vi "FPGA_CounterWriteTimerConfiguration.vi"(6 "UpdateWhenEmpty":bool=TRUE, 8 "error in (no error)":errorcluster, 9 "Average Size":u8=1, 10 "StallPeriod (s)":dbl=0.05, 11 "Ctr Ref in":T1={"DevStatus"={"status"=FALSE, "code"=0, "source"=""}, "CntIndex"=enum."Ctr 1"}) -> (0 "error out":errorcluster, 3 "Ctr Ref out":T1={"DevStatus"={"status"=FALSE, "code"=0, "source"=""}, "CntIndex"=enum."Ctr 1"})   [LabVIEW 2017]
uses:
  <vilib>/Rock Robotics/SystemInterfaces/Counter/FPGA_CounterCtrDevRef.ctl
  <vilib>/Rock Robotics/SystemInterfaces/Counter/FPGA_CounterCtrSystemIndex.ctl
  <vilib>/Rock Robotics/SystemInterfaces/System/FPGA_SystemFPGA Ref Global.vi
  <vilib>/Utility/error.llb/Error Cluster From Error Code.vi
  <vilib>/rvi/errors/niLvFpgaAdjustHostInterfaceError.vi
  <vilib>/rvi/interface/nirviReadWriteControl/nirviReadWriteControl.xnode
  <vilib>/Rock Robotics/SystemInterfaces/System/FPGA_SystemFRC FPGA Ref.ctl
  NiFpgaLv.dll
  <vilib>/rvi/interface/Simulation/niFpgaSimulationCallBeginRW.vi
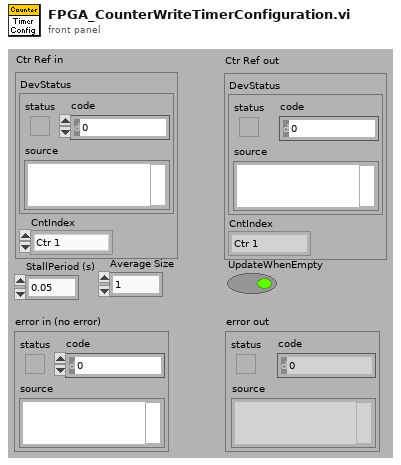
[diagram p1: front panel]
types:
  T1 = typedef "FPGA_CounterCtrDevRef.ctl" = cluster{"DevStatus":errorcluster, "CntIndex":T2}
  T2 = typedef "FPGA_CounterCtrSystemIndex.ctl" = enum8{"Ctr 0", "Ctr 1", "Ctr 2", "Ctr 3", "Ctr 4", "Ctr 5", "Ctr 6", "Ctr 7", "Invalid"}
  T3 = typedef "FPGA_SystemFRC FPGA Ref.ctl" = refnum<k20>
  T4 = cluster{"StallPeriod":fxp<+,24,25>, "AverageSize":fxp<+,7,7>, "UpdateWhenEmpty":bool}
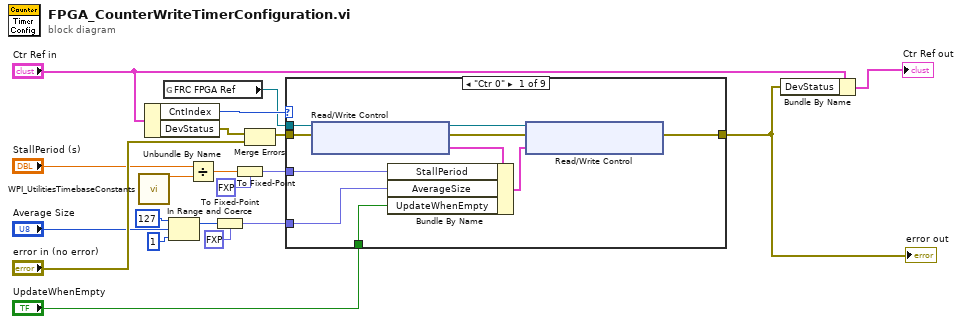
[diagram p0: block diagram]
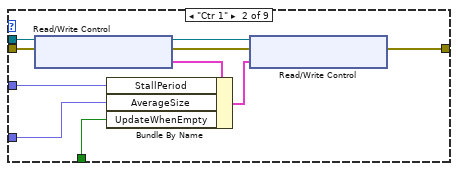
[diagram p2: hidden frame]
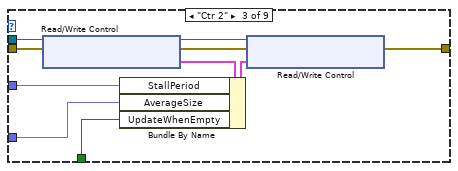
[diagram p3: hidden frame]
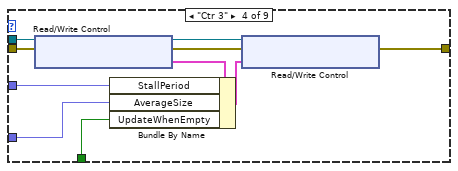
[diagram p4: hidden frame]
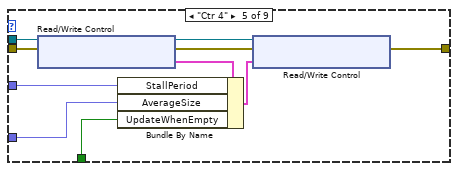
[diagram p5: hidden frame]
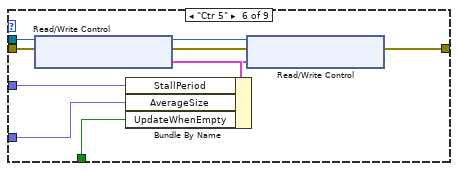
[diagram p6: hidden frame]
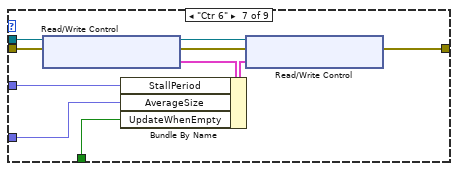
[diagram p7: hidden frame]
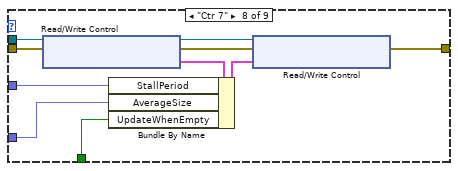
[diagram p8: hidden frame]
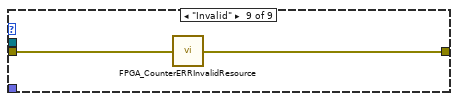
[diagram p9: hidden frame]
diagram:
  n1 = call <vilib>:"WPI_UtilitiesTimebaseConstants.vi"() -> ("40 MHz FPGA clock"=w1:dbl)  [unwired: 13 in, 2 out]
  n2 = Unbundle By Name("Ctr Ref in") -> ("CntIndex"=w14:T2, "DevStatus"=w4:errorcluster)
  n3 = global read "FPGA_SystemFPGA Ref Global.vi" "FRC FPGA Ref"() -> (w3:T3)
  n4 = In Range and Coerce(upper limit=u8 127, x="Average Size", lower limit=u8 1) -> (coerced(x)=w9:u8)  [unwired: 1 out]
  n5 = Divide(x="StallPeriod (s)", y=w1) -> (x/y=w13:dbl)
  n6 = To Fixed-Point(fixed-point type=fxp<+,7,7> 0.0 ("AverageSize"), number=w9) -> (fixed-point=w8:fxp<+,7,7>)
  n7 = To Fixed-Point(fixed-point type=fxp<+,24,25> 0.0 ("StallPeriod"), number=w13) -> (fixed-point=w12:fxp<+,24,25>)
  n8 = Merge Errors(w4, "error in (no error)") -> (w5:errorcluster)
  n9 = case shown="\"Ctr 0\"" w14 {
    tunnel: w3 -> [w21 w31 w50 w60 w70 w80 w90 w100 _]
    tunnel: w5 -> [w30 w34 w49 w59 w69 w77 w89 w99 w101]
    tunnel: [w27 w38 w46 w56 w66 w76 w86 w96 w102] -> w17
    tunnel: w12 -> [w24 w35 w45 w53 w64 w73 w83 w93 _]
    tunnel: w8 -> [w22 w32 w41 w51 w61 w71 w81 w92 _]
    tunnel: "UpdateWhenEmpty" -> [w23 w33 w42 w52 w62 w72 w82 w91 _]
    frame "Ctr 0" {
      n10 = xnode "Read/Write Control"("FPGA VI Reference In"=w21, "error in"=w30) -> ("FPGA VI Reference Out"=w28:T3, "error out"=w29:errorcluster, "Counter0.TimerConfig"=w26:T4)
      n11 = Bundle By Name(cluster=w26, "StallPeriod"=w24, "AverageSize"=w22, "UpdateWhenEmpty"=w23) -> (w25:T4)
      n12 = xnode "Read/Write Control"("FPGA VI Reference In"=w28, "error in"=w29, "Counter0.TimerConfig"=w25) -> ("error out"=w27:errorcluster)  [unwired: 1 out]
    }
    frame "Ctr 1" {
      n13 = xnode "Read/Write Control"("FPGA VI Reference In"=w31, "error in"=w34) -> ("FPGA VI Reference Out"=w39:T3, "error out"=w40:errorcluster, "Counter1.TimerConfig"=w37:T4)
      n14 = Bundle By Name(cluster=w37, "StallPeriod"=w35, "AverageSize"=w32, "UpdateWhenEmpty"=w33) -> (w36:T4)
      n15 = xnode "Read/Write Control"("FPGA VI Reference In"=w39, "error in"=w40, "Counter1.TimerConfig"=w36) -> ("error out"=w38:errorcluster)  [unwired: 1 out]
    }
    frame "Ctr 2" {
      n16 = xnode "Read/Write Control"("FPGA VI Reference In"=w50, "error in"=w49) -> ("FPGA VI Reference Out"=w48:T3, "error out"=w47:errorcluster, "Counter2.TimerConfig"=w44:T4)
      n17 = Bundle By Name(cluster=w44, "StallPeriod"=w45, "AverageSize"=w41, "UpdateWhenEmpty"=w42) -> (w43:T4)
      n18 = xnode "Read/Write Control"("FPGA VI Reference In"=w48, "error in"=w47, "Counter2.TimerConfig"=w43) -> ("error out"=w46:errorcluster)  [unwired: 1 out]
    }
    frame "Ctr 3" {
      n19 = xnode "Read/Write Control"("FPGA VI Reference In"=w60, "error in"=w59) -> ("FPGA VI Reference Out"=w57:T3, "error out"=w58:errorcluster, "Counter3.TimerConfig"=w55:T4)
      n20 = Bundle By Name(cluster=w55, "StallPeriod"=w53, "AverageSize"=w51, "UpdateWhenEmpty"=w52) -> (w54:T4)
      n21 = xnode "Read/Write Control"("FPGA VI Reference In"=w57, "error in"=w58, "Counter3.TimerConfig"=w54) -> ("error out"=w56:errorcluster)  [unwired: 1 out]
    }
    frame "Ctr 4" {
      n22 = xnode "Read/Write Control"("FPGA VI Reference In"=w70, "error in"=w69) -> ("FPGA VI Reference Out"=w67:T3, "error out"=w68:errorcluster, "Counter4.TimerConfig"=w65:T4)
      n23 = Bundle By Name(cluster=w65, "StallPeriod"=w64, "AverageSize"=w61, "UpdateWhenEmpty"=w62) -> (w63:T4)
      n24 = xnode "Read/Write Control"("FPGA VI Reference In"=w67, "error in"=w68, "Counter4.TimerConfig"=w63) -> ("error out"=w66:errorcluster)  [unwired: 1 out]
    }
    frame "Ctr 5" {
      n25 = xnode "Read/Write Control"("FPGA VI Reference In"=w80, "error in"=w77) -> ("FPGA VI Reference Out"=w79:T3, "error out"=w78:errorcluster, "Counter5.TimerConfig"=w75:T4)
      n26 = Bundle By Name(cluster=w75, "StallPeriod"=w73, "AverageSize"=w71, "UpdateWhenEmpty"=w72) -> (w74:T4)
      n27 = xnode "Read/Write Control"("FPGA VI Reference In"=w79, "error in"=w78, "Counter5.TimerConfig"=w74) -> ("error out"=w76:errorcluster)  [unwired: 1 out]
    }
    frame "Ctr 6" {
      n28 = xnode "Read/Write Control"("FPGA VI Reference In"=w90, "error in"=w89) -> ("FPGA VI Reference Out"=w88:T3, "error out"=w87:errorcluster, "Counter6.TimerConfig"=w84:T4)
      n29 = Bundle By Name(cluster=w84, "StallPeriod"=w83, "AverageSize"=w81, "UpdateWhenEmpty"=w82) -> (w85:T4)
      n30 = xnode "Read/Write Control"("FPGA VI Reference In"=w88, "error in"=w87, "Counter6.TimerConfig"=w85) -> ("error out"=w86:errorcluster)  [unwired: 1 out]
    }
    frame "Ctr 7" {
      n31 = xnode "Read/Write Control"("FPGA VI Reference In"=w100, "error in"=w99) -> ("FPGA VI Reference Out"=w98:T3, "error out"=w97:errorcluster, "Counter7.TimerConfig"=w95:T4)
      n32 = Bundle By Name(cluster=w95, "StallPeriod"=w93, "AverageSize"=w92, "UpdateWhenEmpty"=w91) -> (w94:T4)
      n33 = xnode "Read/Write Control"("FPGA VI Reference In"=w98, "error in"=w97, "Counter7.TimerConfig"=w94) -> ("error out"=w96:errorcluster)  [unwired: 1 out]
    }
    frame "Invalid" {
      n34 = call <vilib>:"FPGA_CounterERRInvalidResource.vi"("error in (no error)"=w101) -> ("error out"=w102:errorcluster)
    }
  }
  "error out" <- w17
  n35 = Bundle By Name(cluster="Ctr Ref in", "DevStatus"=w17) -> (→"Ctr Ref out":T1)
